vi "tynySA_test.vi"() -> ()   [LabVIEW 2012]
uses:
  560bf6a7-6959-490f-92d8-cf437f75cecf.vi
panel:
  in  "VISAリソース名":refnum<visa-resource-name>="COM21"
  out "Spectrum analyzer":T1(graph)
  in  "RF":enum8{"fbeat", "fceo"}(ring)=enum."fceo"
  in  "停止":bool
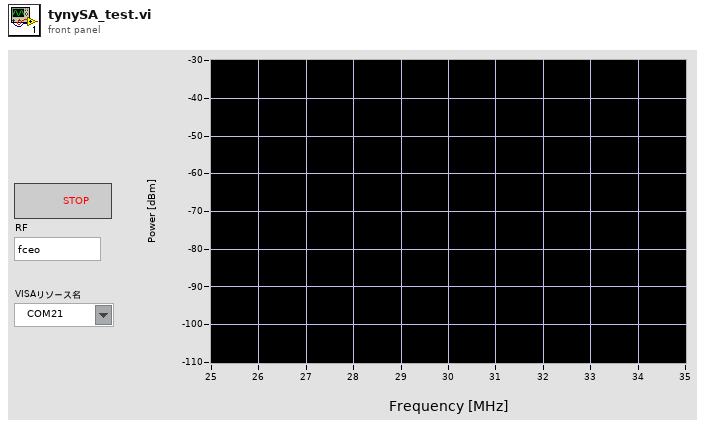
[diagram p1: front panel]
types:
  T1 = cluster{"Frequency (Hz)":dbl[], "Power (dBm)":dbl[]}
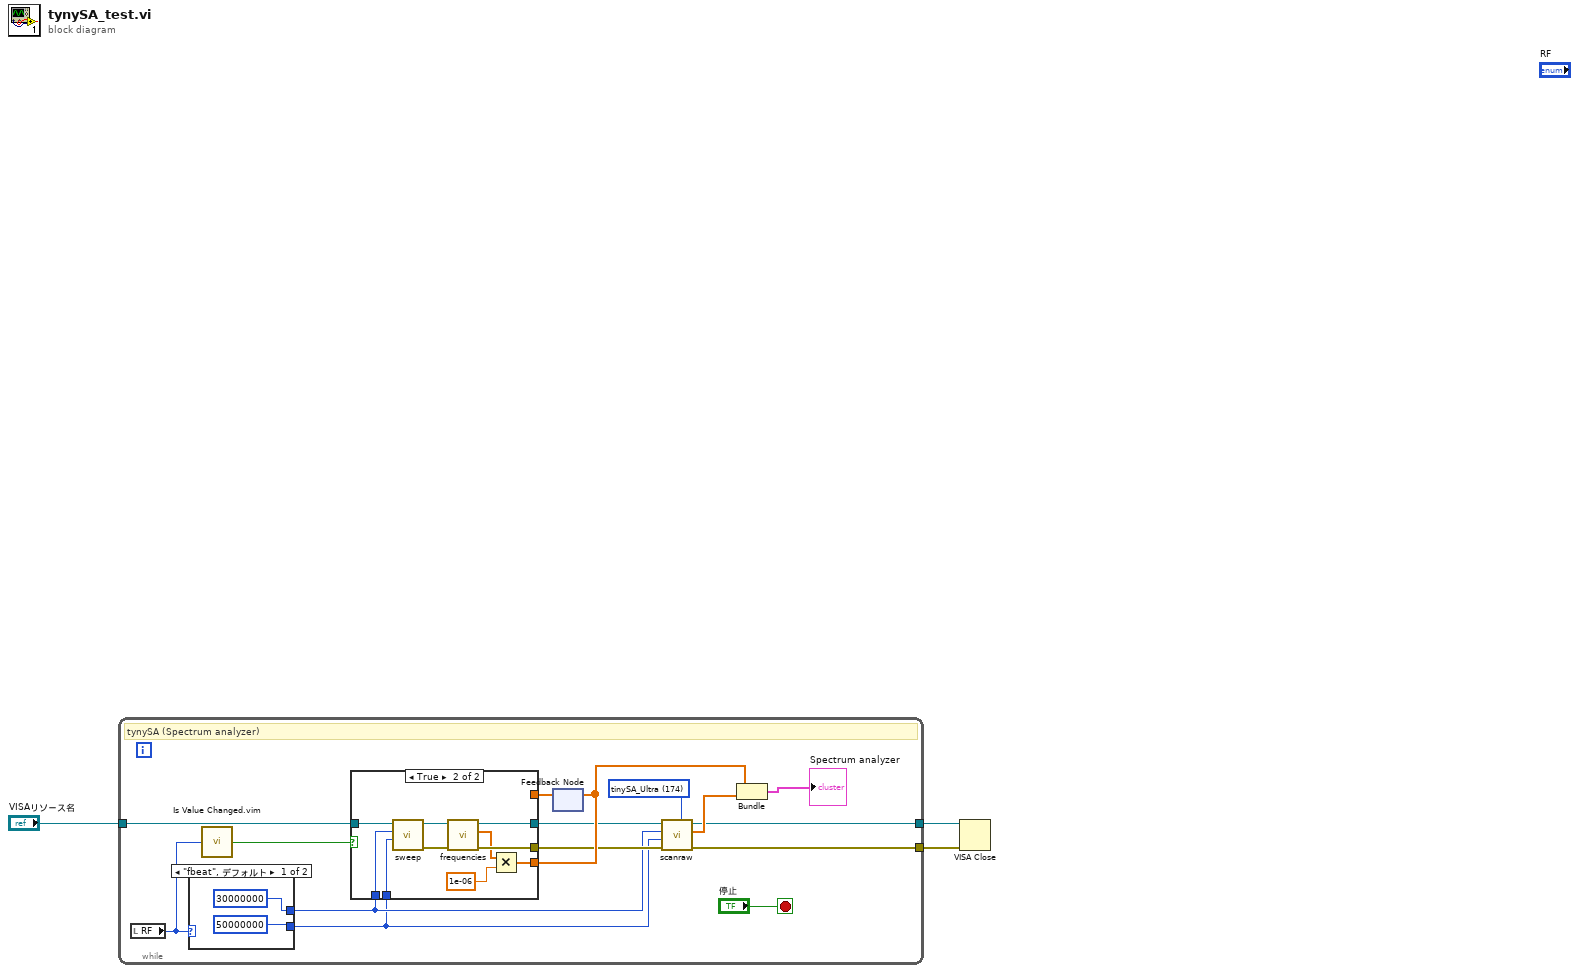
[diagram p0: block diagram]
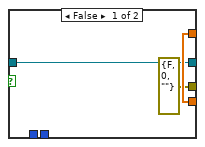
[diagram p2: hidden frame]
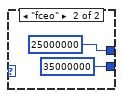
[diagram p3: hidden frame]
diagram:
  n1 = while "Whileループ" {
    tunnel: "VISAリソース名" -> [w10]
    tunnel: [w7] -> w2
    tunnel: [w6] -> w1
    stop <- "停止" stop-if-true
    w18 = u16 174 items=["tinySA"=128, "tinySA_Ultra"=174] ("Offset")
    # "tynySA (Spectrum analyzer)"
    n2 = local read "RF"() -> (w15:enum8{"fbeat", "fceo"})
    n3 = case shown="\"fbeat\", デフォルト" w15 {
      tunnel: [u32 30000000 ("Center Frequency (750 MHz)") u32 25000000 ("Center Frequency (750 MHz)")] -> w5
      tunnel: [u32 50000000 ("Span (1.5 GHz)") u32 35000000 ("Span (1.5 GHz)")] -> w4
      frame "fbeat", Default {
      }
      frame "fceo" {
      }
    }
    n4 = call "Is Value Changed.vim"("value"=w15) -> ("changed or first call?"=w14:bool)
    n5 = feedback #1() -> (w12:dbl[])  [unwired: 1 in]
    n6 = case shown="TRUE" w14 {
      tunnel: [errorcluster {"status"=FALSE, "code"=0, "source"=""} ("Error out") w31] -> w8
      tunnel: [w20 w30] -> w9
      tunnel: [w21 w29] -> w13
      tunnel: w12 -> [w21 _]
      tunnel: w10 -> [w20 w26]
      tunnel: w5 -> [_ w23]
      tunnel: w4 -> [_ w22]
      frame False {
      }
      frame True {
        n7 = call "sweep.vi"("Stop (Hz)"=w22, "Start (Hz)"=w23, "VISA name in"=w26) -> ("Error out"=w24:errorcluster, "VISA name out"=w25:refnum<visa-resource-name>)  [unwired: 7 in]
        n8 = call "frequencies.vi"("Error in"=w24, "VISA name in"=w25) -> ("Error out"=w31:errorcluster, "Frequency (Hz)"=w27:dbl[], "VISA name out"=w30:refnum<visa-resource-name>)  [unwired: 7 in]
        n9 = Multiply(x=w27, y=1e-06 ("scale")) -> (x*y=w29:dbl[])
      }
    }
    n10 = feedback-in #1(w13) -> ()
    n11 = call "scanraw.vi"("Offset"=w18, "Error in"=w8, "Stop (Hz)"=w4, "Start (Hz)"=w5, "VISA name in"=w9) -> ("Error out"=w6:errorcluster, "Power (dBm)"=w17:dbl[], "VISA name out"=w7:refnum<visa-resource-name>)  [unwired: 4 in]
    n12 = Bundle(w13, "Power (dBm)"=w17) -> (→"Spectrum analyzer":cluster{dbl[], "Power (dBm)":dbl[]})  [unwired: 1 in]
  }
  n13 = VISA Close(VISA resource name=w2, error in (no error)=w1) -> ()  [unwired: 1 out]
